vi "Init UI.vi"   [LabVIEW 2020]
uses:
  <vilib>/National Instruments/Tree Map/Tree Map.lvlib
  Scripting/Event types--enum.ctl
  Scripting/DQMH_API.lvlib
types:
  T1 = typedef "Tree Map.lvlib/Tree Map Data.ctl" = map{string, cluster{"Child Paths Set":set{string}, "Name":string, "Data":string, "Attributes":map{string, string}}}
  T2 = typedef "DQMH_API.lvlib/Event types--enum.ctl" = enum16{"Request", "Request and Wait for Reply", "Broadcast"}
  T3 = cluster{"Left Cell String":string, "Child Text":string[], "Child Tag":string, "Item Indent":i32, "Child Only?":bool, "Glyph Index":i32}[]
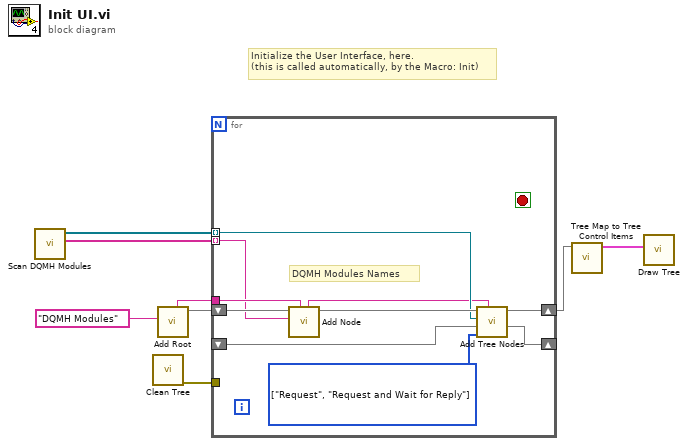
[diagram p0: block diagram]
diagram:
  # "Initialize the User Interface, here.\n(this is called automatically, by the Macro: Init)"
  n1 = call "Scan DQMH Modules.vi"() -> ("Modules List"=w7:string[], "DQMH Modules"=w6:refnum<vi>[])  [unwired: 8 in, 2 out]
  n2 = call "Clean Tree.vi"() -> ("error out"=w8:errorcluster)  [unwired: 11 in]
  n3 = call <vilib>:"Add Root.vi"("New Root Name"="DQMH Modules") -> ("Tree Map Out"=w3:T1, "Root Path"=w4:string)  [unwired: 9 in]
  n4 = for {
    shift-right: [w13] -> w1
    shift-left: w3 -> [w18]
    tunnel: w7 -> [w9] mode=indexing
    tunnel: w4 -> [w17]
    tunnel: w6 -> [w11] mode=indexing
    shift-right: [w14] -> _
    shift-left: _ -> [w15]
    tunnel: w8 -> [_]
    stop <- _ stop-if-true
    w12 = T2[] [enum."Request", enum."Request and Wait for Reply"] items=["Request", "Request and Wait for Reply", "Broadcast"] ("Event Types")
    # "DQMH Modules Names"
    n5 = call <vilib>:"Add Node.vi"("Parent Path"=w17, "New Node Name"=w9, "Tree Map In"=w18) -> ("Tree Map Out"=w16:T1, "New Node Path"=w10:string)  [unwired: 6 in, 1 out]
    n6 = call "Add Tree Nodes.vi"("Root path"=w10, "Event Types"=w12, "map ref in"=w15, "DQMH Lib In"=w11, "Tree Map in"=w16) -> ("map ref out"=w14:map{string, refnum<vi>}, "Tree Map out"=w13:T1)  [unwired: 5 in]
  }
  n7 = call <vilib>:"Tree Map to Tree Control Items.vi"("Tree Map In"=w1) -> ("Tree Control Items"=w5:T3)  [unwired: 10 in]
  n8 = call "Draw Tree.vi"("Tree Control Items"=w5) -> ()  [unwired: 10 in, 1 out]
